vi "VA CoAP Client.vi"() -> (3 "Cancelled?":bool)   [LabVIEW 2020]
doc: "Use this template to create a dialog box with event handling."
panel:
  in  "Token":string
  in  "Message ID":u16=8878 format="%x"
  in  "Method Code":u8(ring)=1 items=["EMPTY", "GET", "POST", "PUT", "DELETE"]
  in  "Type":u8(ring) items=["CONfimable", "NON-confirmable", "ACKnowledgement", "ReSeT"]
  out "New CoAP Message":u8[](array[numeric]) format="%02x"
  in  "URI-Path":string(combo)
  out "Plain Content":string
  out "Response 5":u8 format="%08x"
  out "(hi.lo)":u16
  out "Response 4":u8 format="%08x"
  out "Response 3":u8 format="%08b"
  out "Response 2":u8 format="%08b"
  out "Response 1":u8 format="%08b"
  out "Response 0":u8 format="%08b"
  out "Message to CoAP Server":string
  out "Net address":u32
  out "Reported Address Str":string
  out "Reported Address":u32
  in  "Port":u16(ring)=5683 items=["80"=80, "5683"=5683]
  in  "CoAP Server Address":string(combo)
  out "error out":errorcluster
  out "Response from CoAP Server":string
  in  "Cancel":bool
  in  "OK":bool
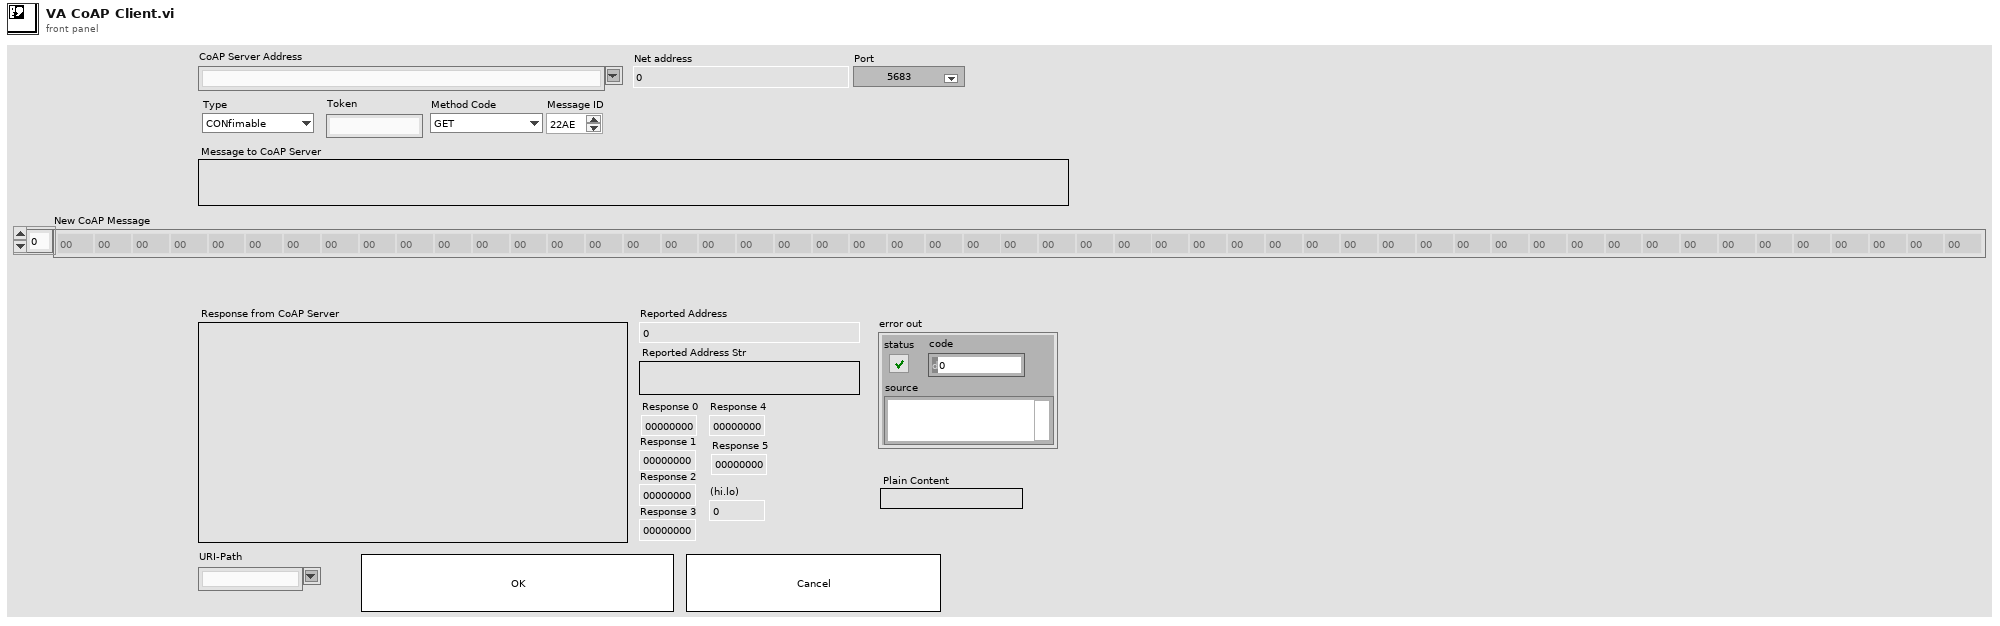
[diagram p1: front panel]
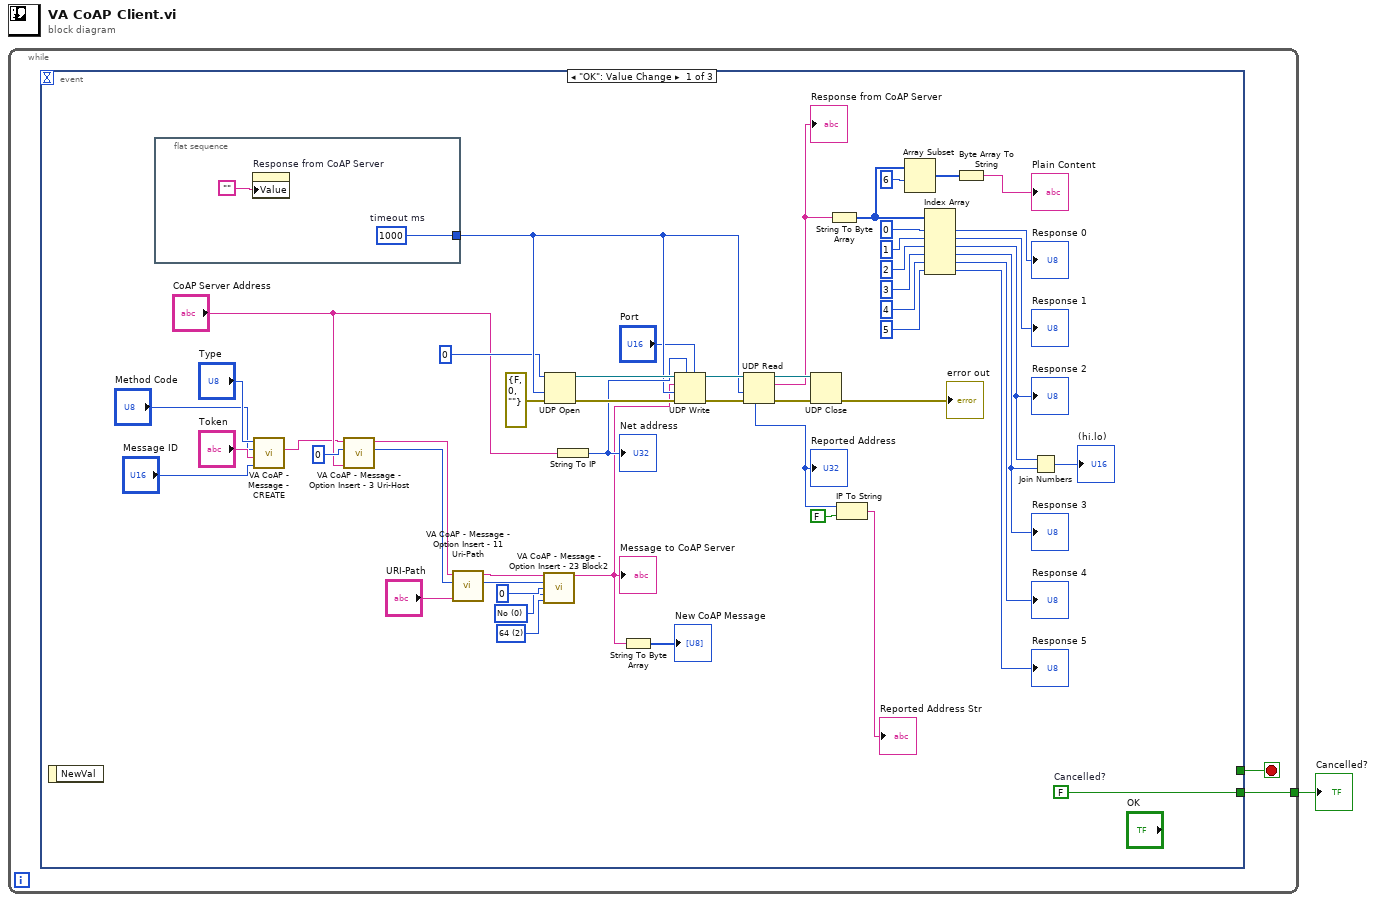
[diagram p0: block diagram]
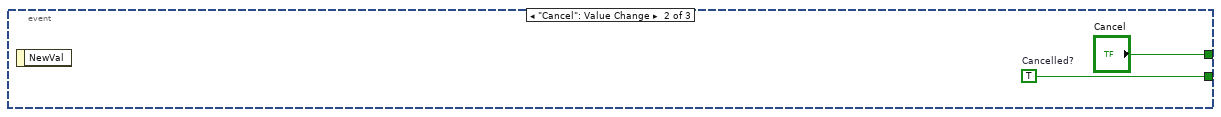
[diagram p2: hidden frame]
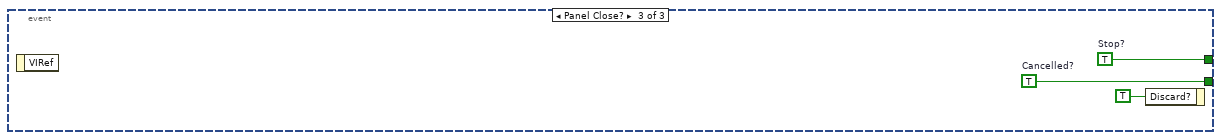
[diagram p3: hidden frame]
diagram:
  n1 = while {
    tunnel: [w2] -> w1
    stop <- w3 stop-if-true
    n2 = event shown="[0] \"OK\": Value Change" {
      selector: _ -> [_ _ _]
      dyn-events: _ -> [_ _ _]
      timeout: _ -> [_ _ _]
      tunnel: [_ "Cancel" w60] -> w3
      tunnel: [w54 w58 w59] -> w2
      event "OK": Value Change {
        w7 = u8 2 items=["16", "32", "64", "128", "256", "512", "1024"] ("SZX (block size)")
        w8 = u8 0 items=["No", "Yes"] ("M (more blocks flag)")
        w54 = FALSE  # Cancelled?
        n3 = event-data() -> ()  [unwired: 1 in, 1 out]
        n4 = flat-sequence {
          tunnel: [w56] -> w42
          frame #0 {
            w56 = 1000  # timeout ms
            n5 = property on="Response from CoAP Server" class="Str"("Value"="") -> ()  [unwired: 2 in, 2 out]
          }
        }
        n6 = call "VA CoAP - Message - CREATE.vi"("Message ID"="Message ID", "Token"="Token", "Method Code"="Method Code", "Type"="Type") -> ("CoAP Message"=w4:string)  [unwired: 6 in]
        n7 = call "VA CoAP - Message - Option Insert - 3 Uri-Host.vi"("CoAP Server Address"="CoAP Server Address", "Current Option Delta"=u8 0, "CoAP Message IN"=w4) -> ("New Option Delta"=w14:u8, "CoAP Message OUT"=w15:string)  [unwired: 6 in]
        n8 = call "VA CoAP - Message - Option Insert - 11 Uri-Path.vi"("URI-Path"="URI-Path", "Current Option Delta"=w14, "CoAP Message IN"=w15) -> ("New Option Delta"=w10:u8, "CoAP Message OUT"=w12:string)  [unwired: 6 in]
        n9 = call "VA CoAP - Message - Option Insert - 23 Block2.vi"("CoAP Message IN"=w12, "Current Option Delta"=w10, "NUM (incremental block number within original data)"=u8 0, "M (more blocks flag)"=w8, "SZX (block size)"=w7) -> ("CoAP Message OUT"=w11:string)  [unwired: 9 in, 1 out]
        "Message to CoAP Server" <- w11
        n10 = UDP Open(8:errorcluster {"status"=FALSE, "code"=0, "source"=""} ("error in (no error)"), 9:w42, 11:u16 0 ("port")) -> (port=w50:refnum<k16>, 0:w48:errorcluster)  [unwired: 2 in, 1 out]
        n11 = String To IP(1:"CoAP Server Address") -> (0:w43:u32)
        "Net address" <- w43
        n12 = String To Byte Array(string=w11) -> (unsigned byte array=→"New CoAP Message":u8[])
        n13 = UDP Write(address=w43, port or service name="Port", connection ID=w50, data in=w11, 8:w48, 9:w42) -> (error out=w47:errorcluster, 3:w49:refnum<k16>)
        n14 = UDP Read(connection ID=w49, timeout ms (25000)=w42, 8:w47) -> (data out=w39:string, error out=w52:errorcluster, 3:w53:refnum<k16>, 6:w46:u32)  [unwired: 1 in, 1 out]
        "Response from CoAP Server" <- w39
        "Reported Address" <- w46
        n15 = UDP Close(connection ID=w53, 8:w52) -> (error out=→"error out":errorcluster)  [unwired: 1 out]
        n16 = String To Byte Array(string=w39) -> (unsigned byte array=w24:u8[])
        n17 = IP To String(1:FALSE ("dot notation? (F)"), 2:w46) -> (0:→"Reported Address Str":string)
        n18 = Array Subset(array=w24, index=6) -> (w22:u8[])  [unwired: 1 in]
        n19 = Index Array(array=w24, index #1=0 ("index"), index #2=1 ("index"), index #3=2 ("index"), index #4=3 ("index"), index #5=4 ("index"), index #6=5 ("index")) -> (element #1=→"Response 0":u8, element #2=→"Response 1":u8, element #3=w29:u8, element #4=w28:u8, element #5=→"Response 4":u8, element #6=→"Response 5":u8)
        "Response 2" <- w29
        "Response 3" <- w28
        n20 = Byte Array To String(unsigned byte array=w22) -> (string=→"Plain Content":string)
        n21 = Join Numbers(hi=w29, lo=w28) -> ((hi.lo)=→"(hi.lo)":u16)
      }
      event "Cancel": Value Change {
        w58 = TRUE  # Cancelled?
        n22 = event-data() -> ()  [unwired: 1 in, 1 out]
      }
      event Panel Close? {
        w59 = TRUE  # Cancelled?
        w60 = TRUE  # Stop?
        n23 = event-data() -> ()  [unwired: 1 in, 1 out]
        n24 = event-data("Discard?"=TRUE) -> ()  [unwired: 1 in, 1 out]
      }
    }
  }
  "Cancelled?" <- w1
